vi "Write Range.vi"(8 "error in (no error)":errorcluster, 9 "Exclude Range (F)":bool, 10 "Range":cluster{"Upper Limit":dbl, "Lower Limit":dbl}, 11 "Interlock Bool in":refnum<class "Interlock Range.lvclass">) -> (0 "error out":errorcluster, 3 "Interlock Bool out":refnum<class "Interlock Range.lvclass">)   [LabVIEW 2015, in "Interlocks.lvlib" / "Interlock Range.lvclass"]
uses:
  Interlock Range.lvclass
  Interlock Range.lvclass/Interlock Range.ctl
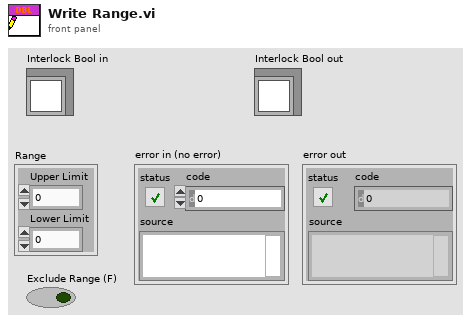
[diagram p1: front panel]
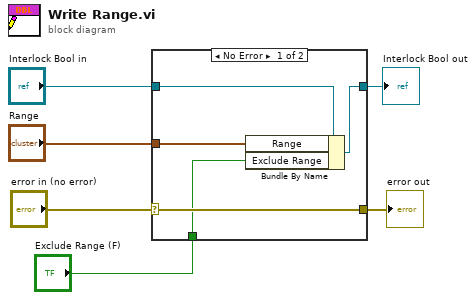
[diagram p0: block diagram]
diagram:
  n1 = case shown="No Error" "error in (no error)" {
    selector: "error in (no error)" -> [w8 w13]
    tunnel: "Interlock Bool in" -> [w11 w12]
    tunnel: [w10 w12] -> w5
    tunnel: "Range" -> [w9 _]
    tunnel: [w8 w13] -> w2
    tunnel: "Exclude Range (F)" -> [w7 _]
    frame No Error {
      n2 = Bundle By Name(cluster=w11, "Range"=w9, "Exclude Range"=w7) -> (w10:refnum<class "Interlock Range.lvclass">)
    }
    frame Error {
    }
  }
  "Interlock Bool out" <- w5
  "error out" <- w2
